vi "Eagle_RT Scanner Control.vi"() -> ()   [LabVIEW 2015]
uses:
  <vilib>/Platform/TimedLoop/XDataNode/timing_clust.ctl
  <vilib>/Platform/TimedLoop/XDataNode/nitl_modes.ctl
  <vilib>/Platform/TimedLoop/XDataNode/wakeup.ctl
  <vilib>/FPGAPlugInAG/cRIO-9030/niLvFpga_Open_cRIO-9030.vi
  <vilib>/rvi/interface/common/dynamic/niFpgaDynamicAddResources.vi
  <vilib>/FPGAPlugInAG/Dynamic/niLvFpga_Run_Dynamic.vi
  <vilib>/Utility/error.llb/Error Cluster From Error Code.vi
  <vilib>/rvi/errors/niLvFpgaAdjustHostInterfaceError.vi
  <vilib>/rvi/interface/nirviOpenFPGA/nirviOpenFPGA.xnode
  FPGA Bitfiles/BELKINEAGLEGUI_FPGATarget_EagleFPGAScanner_FE0ja0MIdO4.lvbitx
  Eagle_FPGA Scanner Control_1.vi
  <vilib>/rvi/interface/nirviMethod/nirviMethod.xnode
  <vilib>/rvi/interface/nirviReadWriteControl/nirviReadWriteControl.xnode
  <vilib>/platform/TimedLoop/XDataNode/XDataNode.xnode
  <vilib>/Platform/TimedLoop/XDataNode/XDNodeRunTimeDep.lvlib
  NiFpgaLv.dll
  <vilib>/rvi/interface/Simulation/niFpgaSimulationCallBeginRW.vi
panel:
  in  "NumOfPoints":i32=100
  in  "Limbus Radius":fxp<+/-,10,10>=250.0
  in  "Limbus Center":T1={"CX"=400.0, "CY"=300.0}
  in  "Center":cluster{"CX":fxp<+,10,10>, "CY":fxp<+,10,10>}
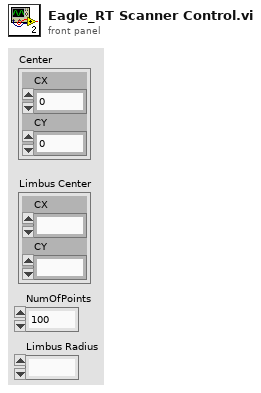
[diagram p1: front panel]
types:
  T1 = cluster{"CX":fxp<+/-,10,10>, "CY":fxp<+/-,10,10>}
  T2 = typedef "XDNodeRunTimeDep.lvlib/timing_clust.ctl" = cluster{"Expected End [f-1]":u64, "Actual End [f-1]":u64, "Finished Late? [f-1]":bool, "Expected End [i-1]":u64, "Actual End [i-1]":u64, "Finished Late? [i-1]":bool, "Expected Start [i]":u64, "Actual Start [i]":u64, "Expected Start [f]":u64, "Actual Start [f]":u64, "Source Name":string, "Structure Name":string, "Period":i64, "Deadline":i64, "Offset":i64, "Start":i64, "Priority":i32, "Timeout":i32, "Mode":T3, "Wakeup Reason":T4, "Error":errorcluster, "Source Type":string, "Secondary Source Type":string, "Global End Time":u64, "Global Start Time":u64, "Frame Duration":u64, "Iteration Duration":u64, "Assigned CPU":i32, "I/O Scan Engine Mode":u32}
  T3 = typedef "XDNodeRunTimeDep.lvlib/nitl_modes.ctl" = enum32{"No Change", "Process missed periods, maintain original phase", "Discard missed periods, maintain original phase", "Process missed periods, ignore original phase", "Discard missed periods, ignore original phase"}
  T4 = typedef "XDNodeRunTimeDep.lvlib/wakeup.ctl" = enum32{"Normal", "Aborted", "Asynchronous wakeup", "Timing source error", "Timed loop error", "Timeout"}
  T5 = cluster{"PxMin":fxp<+,10,10>, "PxMax":fxp<+,10,10>, "PyMin":fxp<+,10,10>, "PyMax":fxp<+,10,10>}
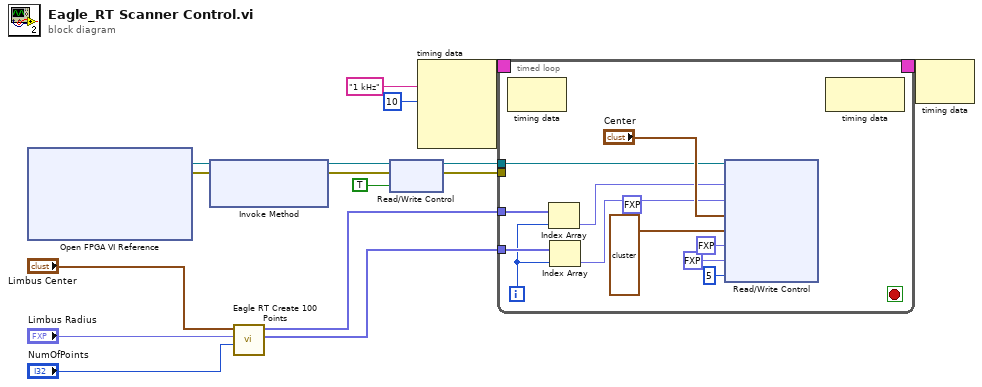
[diagram p0: block diagram]
diagram:
  n1 = xnode "Open FPGA VI Reference"() -> ("FPGA VI Reference Out"=w16:refnum<k20>, "error out"=w15:errorcluster)  [unwired: 2 in]
  n2 = xnode "Invoke Method"("FPGA VI Reference In"=w16, "error in"=w15) -> ("FPGA VI Reference Out"=w10:refnum<k20>, "error out"=w9:errorcluster)  [unwired: 1 in]
  n3 = call "Eagle RT Create 100 Points.vi"("NumOfPoints"="NumOfPoints", "Radius"="Limbus Radius", "Center"="Limbus Center") -> ("PY"=w1:fxp<+,10,10>[], "PX"=w2:fxp<+,10,10>[])  [unwired: 7 in]
  n4 = xnode "Read/Write Control"("FPGA VI Reference In"=w10, "error in"=w9, "Reset"=TRUE) -> ("FPGA VI Reference Out"=w6:refnum<k20>, "error out"=w7:errorcluster)
  n5 = node-c288("1 kHz" ("Source Name"), i64 10 ("Period")) -> (w14:T2)  [unwired: 2 in]
  n6 = timed-loop {
    timing: w14 -> [_]
    timing-out: [_] -> w13
    tunnel: w7 -> [_]
    tunnel: w6 -> [w22]
    tunnel: w2 -> [w21]
    tunnel: w1 -> [w20]
    i -> [w19]
    stop <- _ stop-if-true
    (unwired) fxp<+/-,10,10> 0.0 ("element")
    n7 = node-c288() -> ()  [unwired: 1 in, 1 out]
    n8 = Index Array(array=w21, index=w19) -> (element=w18:fxp<+,10,10>)
    n9 = Index Array(array=w20, index=w19) -> (element=w17:fxp<+,10,10>)
    n10 = xnode "Read/Write Control"("FPGA VI Reference In"=w22, "PX"=w18, "PY"=w17, "Center"="Center", "NoGO Zone"=T5 {"PxMin"=300.0, "PxMax"=500.0, "PyMin"=200.0, "PyMax"=400.0}, "VX OFFS"=fxp<+/-,16,1> 0.0, "VY OFFS"=fxp<+/-,16,1> 0.0, "NumOfRetries"=u16 5) -> ()  [unwired: 1 in, 2 out]
    n11 = node-c288() -> ()  [unwired: 1 in, 1 out]
  }
  n12 = node-c288(w13) -> ()  [unwired: 1 out]
